vi "InitTimeOfFlightSensors.vi"(8 "error in (no error)":errorcluster, 9 "Multi ToF Config":T1={"I2C Channel"=1, "Number of Sensors"=4, "Sensor Relay DIO Pins"=[16, 17, 18, 19]}, 11 "LINX Resource":T3) -> (0 "error out":errorcluster, 1 "VL6180 Resources":T2[](array[typedef]) {"I2C Slave Address" format="%02x"}, 2 "ToFOnline":bool[](array[boolean]), 3 "LINX Resource Out":T3)   [LabVIEW 2014]
uses:
  <vilib>/MakerHub/LINX/Private/Type Defs/LINX Ref.ctl
  <vilib>/MakerHub/LINX/Private/Type Defs/Platform.ctl
  <vilib>/MakerHub/LINX/Private/Type Defs/Interface.ctl
  <vilib>/MakerHub/LINX/Private/Device/Type Defs/LINX Device Config.ctl
  <vilib>/MakerHub/LINX/Private/Device/Type Defs/TCP Config.ctl
  <vilib>/MakerHub/LINX/Private/Device/Type Defs/Channels.ctl
  Sensors/Time of Flight - VL6180/VL6180 Resource.ctl
  <vilib>/MakerHub/LINX/Public/Peripherals/Digital/Digital Write 1 Chan.vi
  <vilib>/MakerHub/LINX/Public/Peripherals/Digital/Digital Write N Chans.vi
  <vilib>/MakerHub/LINX/Private/Local IO/LinxDigitalWrite.vi
  <vilib>/MakerHub/LINX/Public/Utilities/Check Channel.vi
  <vilib>/myRIO/Instrument Drivers/Onboard IO/DIO/vis/Write.vi
  <vilib>/MakerHub/LINX/Private/myRIO/Utilities/Get DIO Channel Name.vi
  <vilib>/MakerHub/LINX/Private/Utilties/Generate Error.vi
  <vilib>/myRIO/Instrument Drivers/Onboard IO/DIO/vis/Smart Open.vi
  <vilib>/Utility/error.llb/Error Cluster From Error Code.vi
  <vilib>/myRIO/Common/Instrument Driver Framework/myRIO v1.0/DIO/vis/myRIO v1.0 Write DIO.vi
  <vilib>/MakerHub/LINX/LMH-LINX.lvlib
  <vilib>/MakerHub/LINX/Private/Device/Device.lvlib
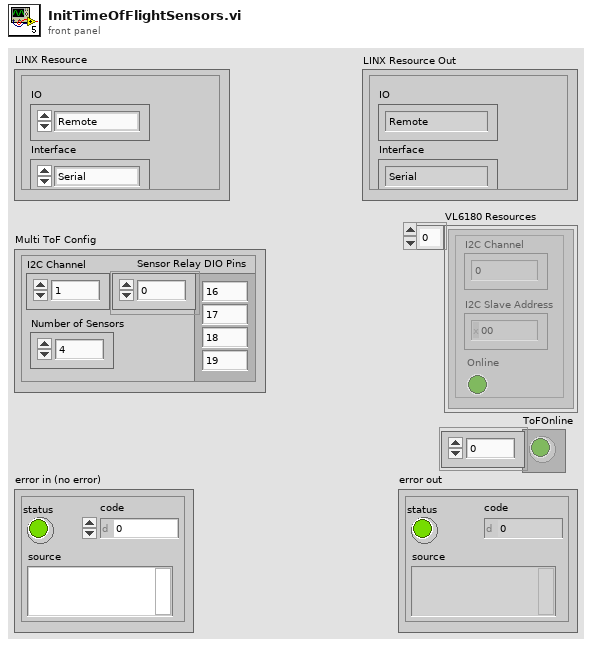
[diagram p1: front panel]
types:
  T1 = cluster{"I2C Channel":u8, "Number of Sensors":u8, "Sensor Relay DIO Pins":u8[]}
  T2 = typedef "VL6180 Resource.ctl" = cluster{"I2C Channel":u8, "I2C Slave Address":u8, "Online":bool}
  T3 = typedef "LMH-LINX.lvlib/LINX Ref.ctl" = cluster{"IO":T4, "Interface":T5, "LINX Device Config":T6}
  T4 = typedef "LMH-LINX.lvlib/Platform.ctl" = enum16{"Remote", "Local"}
  T5 = typedef "LMH-LINX.lvlib/Interface.ctl" = enum16{"Serial", "TCP"}
  T6 = typedef "LMH-LINX.lvlib/Device.lvlib/LINX Device Config.ctl" = cluster{"Interface":T5, "COM Port":refnum<visa-resource-name>, "TCP Configuration":T7, "Device Family":u8, "Device ID":u8, "Device Name":string, "TCP Ref":refnum<k5>, "Channels":T8}
  T7 = typedef "LMH-LINX.lvlib/Device.lvlib/TCP Config.ctl" = cluster{"IP Address":string, "Port":u16}
  T8 = typedef "LMH-LINX.lvlib/Channels.ctl" = cluster{"DI":u8[], "DO":u8[], "AI":u8[], "AO":u8[], "PWM":u8[], "QE":u8[], "UART":u8[], "I2C 2":u8[], "SPI":u8[], "CAN":u8[], "Servo":u8[], "AI Ref (V)":dbl, "AI Resolution (Bits)":u8, "AO Ref (V)":dbl, "AO Resolution (Bits)":u8}
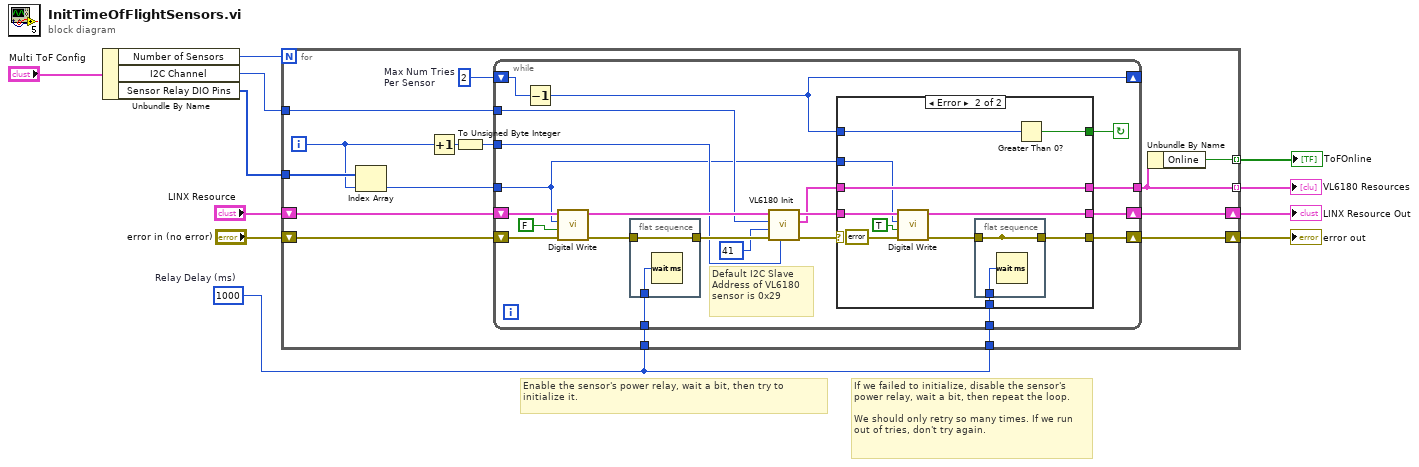
[diagram p0: block diagram]
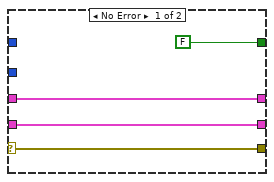
[diagram p2: hidden frame]
diagram:
  w8 = u32 1000  # Relay Delay (ms)
  # "If we failed to initialize, disable the sensor's power relay, wait a bit, then repeat the loop.\n\nWe should only retry so many times. If we run out of tries, don't try again."
  # "Enable the sensor's power relay, wait a bit, then try to initialize it."
  n1 = Unbundle By Name("Multi ToF Config") -> ("Number of Sensors"=w2:u8, "I2C Channel"=w3:u8, "Sensor Relay DIO Pins"=w4:u8[])
  n2 = for {
    N: w2 -> [_]
    tunnel: w3 -> [w21]
    tunnel: w4 -> [w26]
    shift-right: [w19] -> w10
    shift-left: "error in (no error)" -> [w24]
    shift-right: [w18] -> w7
    shift-left: "LINX Resource" -> [w23]
    tunnel: w8 -> [w22]
    tunnel: w8 -> [w20]
    tunnel: [w16] -> w6 mode=indexing
    tunnel: [w15] -> w1 mode=indexing
    i -> [w13]
    w17 = 2  # Max Num Tries Per Sensor
    n3 = Index Array(array=w26, index=w13) -> (element=w25:u8)
    n4 = Increment(x=w13) -> (x+1=w14:i32)
    n5 = To Unsigned Byte Integer(number=w14) -> (unsigned 8bit integer=w12:u8)
    n6 = while {
      tunnel: w25 -> [w27]
      shift-right: [w34] -> w18
      shift-left: w23 -> [w47]
      shift-right: [w33] -> w19
      shift-left: w24 -> [w46]
      tunnel: w22 -> [w43]
      tunnel: w21 -> [w38]
      tunnel: w12 -> [w40]
      tunnel: w20 -> [w35]
      tunnel: [w32] -> w16
      shift-right: [w29] -> _
      shift-left: w17 -> [w31]
      stop <- w30 continue-if-true
      # "Default I2C Slave Address of VL6180 sensor is 0x29"
      n7 = Decrement(x=w31) -> (x-1=w29:i32)
      n8 = call-poly <vilib>:"Digital Write.vi"("Error In"=w46, "Output Value"=FALSE, "DO Channel"=w27, "LINX Resource"=w47) -> ("Error Out"=w44:errorcluster, "LINX Resource"=w41:T3)  [unwired: 6 in]
      n9 = flat-sequence {
        tunnel: [w66] -> w42
        tunnel: w44 -> [w66]
        tunnel: w43 -> [w65]
        frame #0 {
          n10 = Wait (ms)(milliseconds to wait=w65) -> ()  [unwired: 1 out]
        }
      }
      n11 = call "VL6180 Init.vi"("Change Slave Address"=w40, "Error In"=w42, "I2C Slave Address"=u8 41 ("I2C Slave Address (0)"), "I2C Channel"=w38, "LINX Resource"=w41) -> ("Error Out"=w37:errorcluster, "VL6180 Resource"=w28:T2, "LINX Resource"=w36:T3)  [unwired: 4 in]
      n12 = case shown="Error" w37 {
        selector: w37 -> [w50 _]
        tunnel: w36 -> [w51 w62]
        tunnel: w35 -> [_ w60]
        tunnel: [w51 w59] -> w34
        tunnel: [w50 w58] -> w33
        tunnel: w28 -> [w49 w56]
        tunnel: [w49 w56] -> w32
        tunnel: [FALSE w55] -> w30
        tunnel: w29 -> [_ w54]
        tunnel: w27 -> [_ w53]
        frame No Error {
        }
        frame Error {
          n13 = call-poly <vilib>:"Digital Write.vi"("Error In"=errorcluster {"status"=FALSE, "code"=0, "source"=""}, "Output Value"=TRUE, "DO Channel"=w53, "LINX Resource"=w62) -> ("Error Out"=w61:errorcluster, "LINX Resource"=w59:T3)  [unwired: 6 in]
          n14 = flat-sequence {
            tunnel: [w63] -> w58
            tunnel: [w63] -> _
            tunnel: w60 -> [w64]
            tunnel: w61 -> [w63]
            frame #0 {
              n15 = Wait (ms)(milliseconds to wait=w64) -> ()  [unwired: 1 out]
            }
          }
          n16 = Greater Than 0?(x=w54) -> (x > 0?=w55:bool)
        }
      }
    }
    n17 = Unbundle By Name(w16) -> ("Online"=w15:bool)
  }
  "error out" <- w10
  "LINX Resource Out" <- w7
  "VL6180 Resources" <- w6
  "ToFOnline" <- w1
